vi "Read Voltage.vi"(8 "error in (no error)":errorcluster, 11 "Virtual Voltmeter in":refnum<class "Virtual Voltmeter.lvclass">) -> (0 "error out":errorcluster, 2 "Voltage":dbl format="%#_g V", 3 "Virtual Voltmeter out":refnum<class "Virtual Voltmeter.lvclass">)   [LabVIEW 2023, in "Voltmeter.lvlib" / "Virtual Voltmeter.lvlib" / "Virtual Voltmeter.lvclass"]
uses:
  Virtual Voltmeter.lvclass
  Virtual Voltmeter.lvclass/Virtual Voltmeter.ctl
  Interfaces/IRead Voltage Multichannel/IRead Voltage from Channel.lvclass
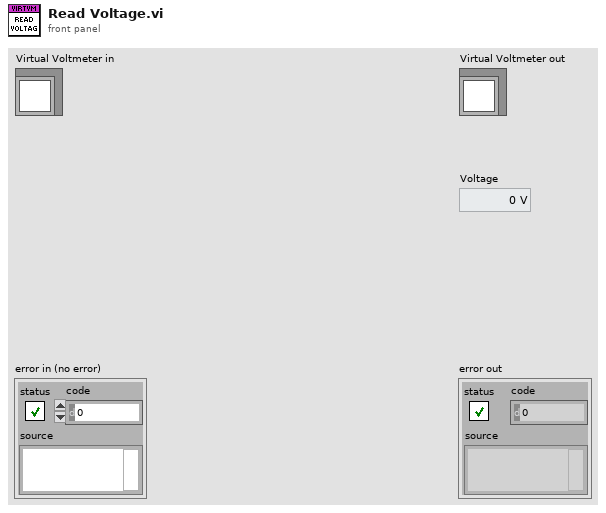
[diagram p1: front panel]
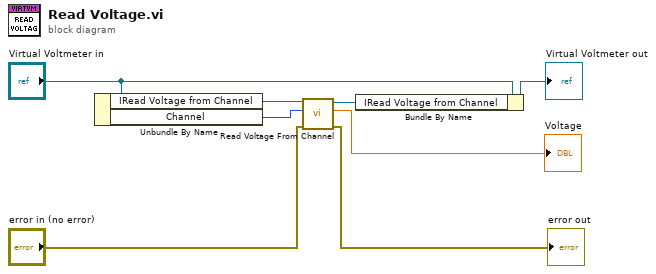
[diagram p0: block diagram]
diagram:
  n1 = Unbundle By Name("Virtual Voltmeter in") -> ("IRead Voltage from Channel"=w7:refnum<class "IRead Voltage from Channel.lvclass">, "Channel"=w4:u8)
  n2 = call-dynamic "Read Voltage From Channel.vi"("error in (no error)"="error in (no error)", "Channel"=w4, "IRead Voltage Multichannel in"=w7) -> ("error out"=→"error out":errorcluster, "Voltage"=→"Voltage":dbl, "IRead Voltage Multichannel out"=w1:refnum<class "IRead Voltage from Channel.lvclass">)  [unwired: 6 in]
  n3 = Bundle By Name(cluster="Virtual Voltmeter in", "IRead Voltage from Channel"=w1) -> (→"Virtual Voltmeter out":refnum<class "Virtual Voltmeter.lvclass">)
